vi "Main_FGV.vi"() -> ()   [LabVIEW 2018]
uses:
  Control/serial.ctl
  F:/Program Files (x86)/National Instruments/LabVIEW 2018/examples/Instrument IO/Serial/support/Serial - Settings.ctl
panel:
  out "Response":string
  in  "Command":string="*IDN?"
  in  "쓰기?":bool
  in  "Serial Settings":T1={"baud rate"=9600, "data bits"=8, "parity"=enum."None", "stop bits"=10, "flow control"=0} {"flow control" items=["None"=0, "XON/XOFF"=1, "RTS/CTS"=2, "DTR/DSR"=4]; "stop bits" items=["1.0"=10, "1.5"=15, "2.0"=20]; "data bits" min=5 max=8 step=1; "baud rate" items=["75"=75, "110"=110, "134"=134, "150"=150, "300"=300, "600"=600, "1200"=1200, "1800"=1800, "2400"=2400, "4800"=4800, "7200"=7200, "9600"=9600, "14400"=14400, "19200"=19200, "28800"=28800, "38400"=38400, "56000"=56000, "57600"=57600, "115200"=115200, "128000"=128000, "230400"=230400]}
  in  "VISA resource name":refnum<visa-resource-name>="COM1"
  in  "정지":bool
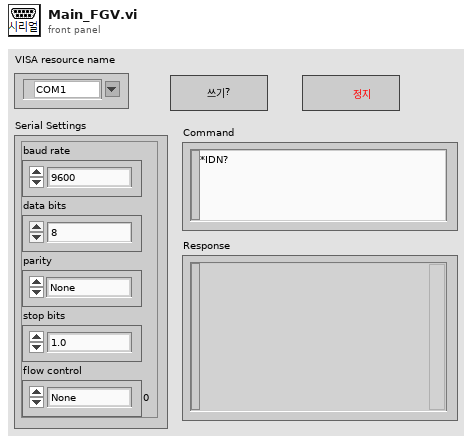
[diagram p1: front panel]
types:
  T1 = typedef "Serial - Settings.ctl" = cluster{"baud rate":u32, "data bits":u16, "parity":enum16{"None", "Odd", "Even", "Mark", "Space"}, "stop bits":u16, "flow control":u16}
  T2 = typedef "serial.ctl" = enum16{"설정", "읽기", "쓰기", "종료"}
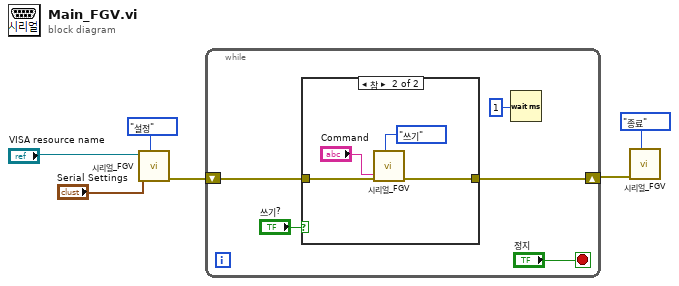
[diagram p0: block diagram]
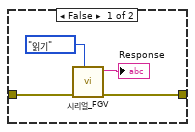
[diagram p2: hidden frame]
diagram:
  n1 = call "시리얼_FGV.vi"("state"=serial."설정", "Serial Settings"="Serial Settings", "VISA resource name"="VISA resource name") -> ("Error Out"=w4:errorcluster)  [unwired: 7 in, 1 out]
  n2 = while {
    shift-right: [w8] -> w3
    shift-left: w4 -> [w9]
    stop <- "정지" stop-if-true
    n3 = case shown="참" "쓰기?" {
      tunnel: w9 -> [w15 w19]
      tunnel: [w14 w17] -> w8
      frame False {
        n4 = call "시리얼_FGV.vi"("state"=serial."읽기", "Error In"=w15) -> ("Error Out"=w14:errorcluster, "Response"=→"Response":string)  [unwired: 8 in]
      }
      frame True {
        n5 = call "시리얼_FGV.vi"("Command"="Command", "state"=serial."쓰기", "Error In"=w19) -> ("Error Out"=w17:errorcluster)  [unwired: 7 in, 1 out]
      }
    }
    n6 = Wait (ms)(milliseconds to wait=u32 1 ("ms 타이머 값")) -> ()  [unwired: 1 out]
  }
  n7 = call "시리얼_FGV.vi"("state"=serial."종료", "Error In"=w3) -> ()  [unwired: 8 in, 2 out]
